vi "Send Roles API.vi"(8 "error in (no error)":errorcluster, 10 "Subscriber":refnum<class "MessageQ.lvclass">, 11 "Role Manager in":refnum<class "Role Manager.lvclass">) -> (0 "error out":errorcluster, 3 "Role Manager out":refnum<class "Role Manager.lvclass">)   [LabVIEW 2020, in "Volatus.lvlib" / "Role Manager.lvclass"]
uses:
  Role Manager.lvclass
  MessageQ/MessageQ.lvclass
  Role Manager.lvclass/Role Manager.ctl
  MessageQ/MessageQ.lvclass/MessageQ.ctl
  Roles API/Roles API.lvclass
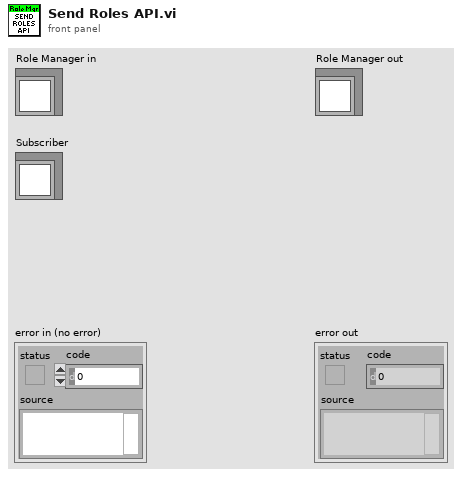
[diagram p1: front panel]
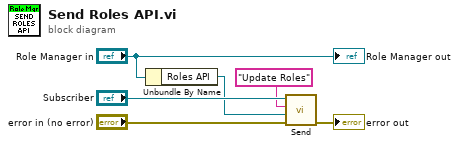
[diagram p0: block diagram]
diagram:
  n1 = Unbundle By Name("Role Manager in") -> ("Roles API"=w4:refnum<class "Roles API.lvclass">)
  n2 = call "Send.vi"("error in (no error)"="error in (no error)", "Data"=w4, "ID"="Update Roles", "MessageQ in"="Subscriber") -> ("error out"=→"error out":errorcluster)  [unwired: 6 in, 1 out]
  "Role Manager out" <- "Role Manager in"
